vi "Actor Core.vi"(8 "error in":errorcluster, 11 "Target Reply Time Test Actor in":refnum<class "Target Reply Time Test Actor.lvclass">) -> (0 "error out":errorcluster, 3 "Actor out":refnum<class "Actor.lvclass">)   [LabVIEW 2023, in "Target Reply Time Test Actor.lvlib" / "Target Reply Time Test Actor.lvclass"]
doc: "(<B>Filename</B>: Actor Framework.lvlib:Actor.lvclass:Actor Core.vi)\n\nReceives messages to the actor, reacts to them, and initiates any error handling that may shut the actor down.\n\nDescendant classes may override this VI to append parallel tasks for the actor to complete while it handles messages. Overrides use the Call Parent Class Method node."
uses:
  Target Reply Time Test Actor.lvclass
  C:/Program Files/National Instruments/LabVIEW 2023/vi.lib/ActorFramework/Actor/Actor.lvclass
  <vilib>/ActorFramework/Actor/Actor.lvclass
  Target Reply Time Test Actor Messages/Reply Msg DataSocket Msg/Reply Msg DataSocket Msg.lvclass
  <vilib>/ni/Actors/Network Endpoint Actors/Notifying Nested Endpoint/Notifying Nested Endpoint.lvclass
  C:/Program Files/National Instruments/LabVIEW 2023/vi.lib/ni/Actors/Network Endpoint Actors/Network Endpoint/Network Endpoint/Network Endpoint.lvclass
  Target Reply Time Test Actor.lvclass/Target Reply Time Test Actor.ctl
  <vilib>/ni/Actors/Network Endpoint Actors/Network Endpoint/Network Endpoint/Network Endpoint.lvclass/Network Endpoint.ctl
  <vilib>/ni/Actors/Network Endpoint Actors/Network Endpoint/Network Endpoint/Network Endpoint.lvclass
  Reply Msg DataSocket/Reply Msg DataSocket.lvclass
  Target Reply Time Test Actor Messages/Shutdown Msg/Shutdown Msg.lvclass
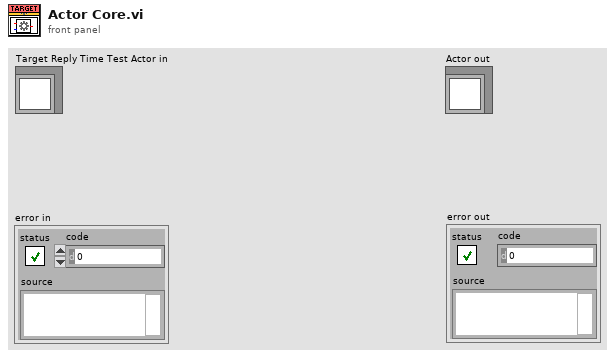
[diagram p1: front panel]
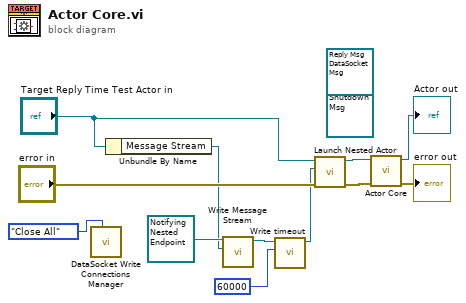
[diagram p0: block diagram]
diagram:
  (unwired) refnum<class "Shutdown Msg.lvclass"> refnum ("Target Reply Time Test Actor.lvlib:Shutdown Msg.lvclass")
  (unwired) refnum<class "Reply Msg DataSocket Msg.lvclass"> refnum ("Target Reply Time Test Actor.lvlib:Reply Msg DataSocket Msg.lvclass")
  n1 = call "DataSocket Write Connections Manager.vi"("Action"=enum16{"Get", "Close", "Close All"}."Close All") -> ()  [unwired: 10 in, 1 out]
  n2 = Unbundle By Name("Target Reply Time Test Actor in") -> ("Message Stream"=w6:refnum<class "Message Stream.lvclass">)
  n3 = call <vilib>:"Write Message Stream.vi"("Message Stream"=w6, "Network Endpoint in"=refnum<class "Notifying Nested Endpoint.lvclass"> refnum ("Notifying Nested Endpoint.lvclass")) -> ("Network Endpoint out"=w7:refnum<class "Notifying Nested Endpoint.lvclass">)  [unwired: 9 in]
  n4 = call <vilib>:"Write timeout.vi"("timeout"=60000, "Network Endpoint in"=w7) -> ("Network Endpoint out"=w2:refnum<class "Notifying Nested Endpoint.lvclass">)  [unwired: 9 in]
  n5 = call <vilib>:"Launch Nested Actor.vi"("error in (no error)"="error in", "Nested Actor"=w2, "Caller Actor in"="Target Reply Time Test Actor in") -> ("error out"=w5:errorcluster, "Caller Actor out"=w4:refnum<class "Target Reply Time Test Actor.lvclass">)  [unwired: 6 in, 1 out]
  n6 = call-parent "Actor Core.vi"("error in"=w5, "Actor in"=w4) -> ("error out"=→"error out":errorcluster, "Actor out"=→"Actor out":refnum<class "Actor.lvclass">)  [unwired: 8 in]
